vi "Main.vi"() -> ()   [LabVIEW 2020, in "ChromTech Next Gen Compensator Pump.lvlib"]
uses:
  ChromTech Next Gen Compensator Pump.lvlib
  process loops/Instrument Manager/Instrument State.ctl
  process loops/UI Manager/Data Display Loop Data.ctl
  process loops/Logging/Logging Configuration.ctl
  process loops/UI Manager/UI Data.ctl
  process loops/UI Manager/UI Display State.ctl
  Typedefs/System Control Data.ctl
  <vilib>/Utility/error.llb/Error Cluster From Error Code.vi
  <vilib>/ErrorRing/Error Ring.xnode
  support/Message Queue/Message Queue.lvlib
  support/User Event - Stop/User Event - Stop.lvlib
  process loops/Instrument Manager/Instrument Manager.lvlib
  process loops/Acquisition/Acquisition.lvlib
  process loops/Remote Connection Manager/Remote Connection Manager.lvlib
  process loops/Logging/Logging.lvlib
panel:
  in  "This Flow Rate (mL/min)":dbl format="%.3f"
  in  "Total Flow (mL/min)":dbl=0.1 format="%.3f"
  in  "Time Interval (sec)":i32=1200
  out "Data Graph":cluster{timestamp[], dbl[]}[](graph)
  in  "Config Log Btn":bool
  in  "Sampling rate\n(sec/sample)":dbl=5.0 min=0.1 step=0.1
  in  "Log Data":bool
  in  "Stop Btn":bool=TRUE
  in  "Run Btn":bool
  out "Data Ind":dbl format="%d psi"
  in  "Other Flow Rate (mL/min)":dbl format="%.3f"
  out "VISA resource":refnum<visa-resource-name>
  # "Pump Control Panel"
  # "Config"
  # "Pump Control"
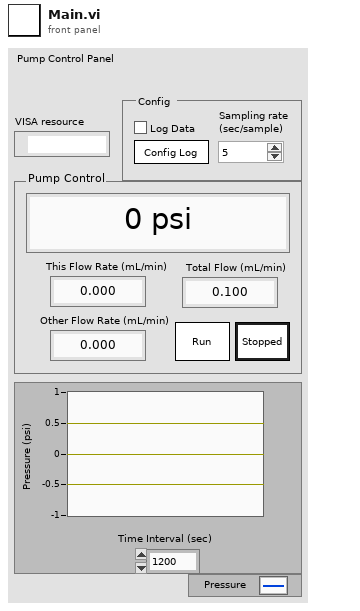
[diagram p1: front panel]
types:
  T1 = typedef "ChromTech Next Gen Compensator Pump.lvlib/Data Display Loop Data.ctl" = cluster{"Data Timestamps":timestamp[], "Data Values":dbl[], "Previous Run State":bool}
  T2 = typedef "ChromTech Next Gen Compensator Pump.lvlib/Instrument Manager.lvlib/Instrument State.ctl" = cluster{"VISA Resource":refnum<visa-resource-name>, "Flow Rate":dbl, "Running":bool, "Running Since":timestamp, "Pressure Data Point":cluster{"Time Stamp":timestamp, "Value":dbl}, "Upper Pressure Fault":bool, "Lower Pressure Fault":bool, "Motor Stall Fault":bool, "Sampling Rate (sec/sample)":dbl, "Retry Attempts":i32, "Fast Comms":bool, "Total Flow Rate":dbl, "Other Flow Rate":dbl}
  T3 = typedef "ChromTech Next Gen Compensator Pump.lvlib/Message Queue.lvlib/All Message Queues.ctl" = cluster{"System Control":refnum<queue>, "Instrument":refnum<queue>, "Remote":refnum<queue>, "UI":refnum<queue>, "Acquisition":refnum<queue>, "Logging":refnum<queue>}
  T4 = typedef "ChromTech Next Gen Compensator Pump.lvlib/UI Display State.ctl" = enum16{"Shown", "Hidden"}
  T5 = enum8{"Enabled", "Disabled", "Disabled and Grayed Out"}
  T6 = typedef "ChromTech Next Gen Compensator Pump.lvlib/UI Data.ctl" = cluster{"VISA Resource Ind":refnum<vi>, "Setpoint Ctl":refnum<vi>, "Run Btn":refnum<vi>, "Stop Btn":refnum<vi>, "Data Ind":refnum<vi>, "Log Data":refnum<vi>, "Config Log Btn":refnum<vi>, "Sampling rate\n(sec/sample)":refnum<vi>, "Data Graph":refnum<vi>, "This Flow Rate (mL/min)":refnum<vi>, "Other Flow Rate (mL/min)":refnum<vi>, "Total Flow (mL/min)":refnum<vi>}
  T7 = typedef "ChromTech Next Gen Compensator Pump.lvlib/Logging.lvlib/Logging Configuration.ctl" = cluster{"Log Directory Path":path, "Log File Path":path, "Log File Prefix":string, "Log File Extension":string, "File Delimiter":string, "Header Info":string[][], "Channels":string[], "Log Instrument Runs":bool}
  T8 = typedef "ChromTech Next Gen Compensator Pump.lvlib/System Control Data.ctl" = cluster{"Example Value <Replace Me>":dbl, "Log Runs":bool, "Clone":bool}
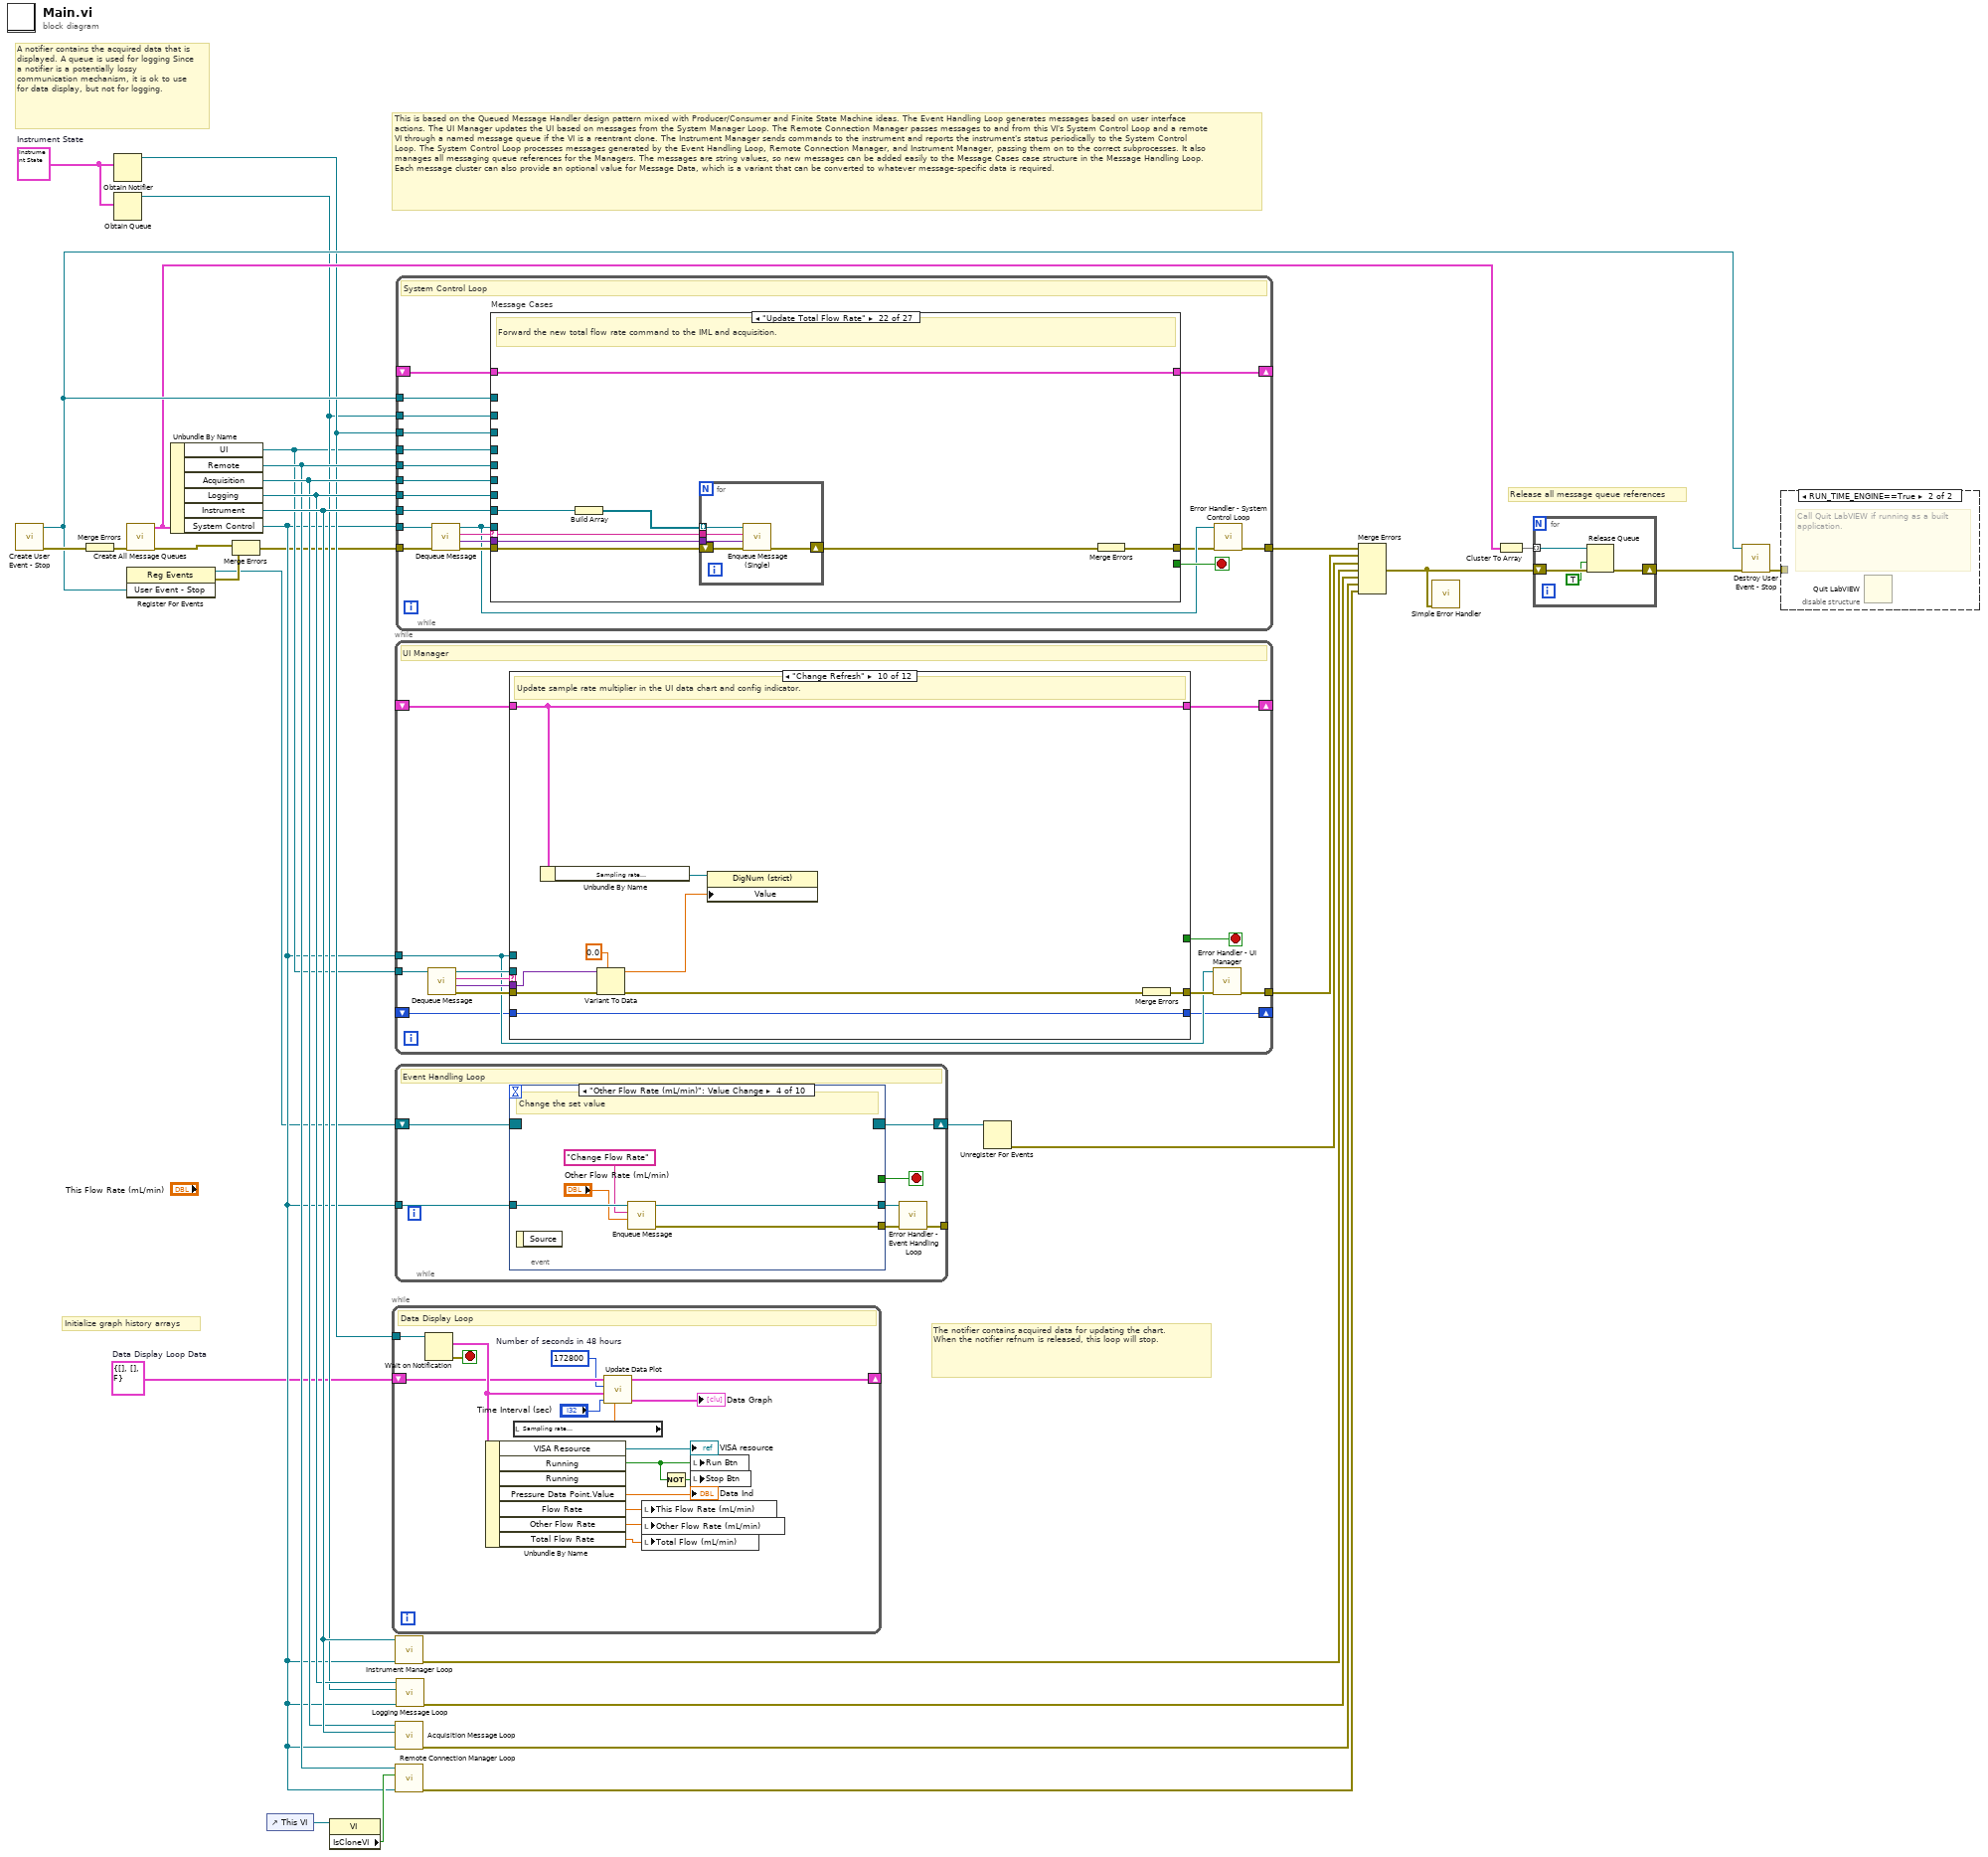
[diagram p0: block diagram]
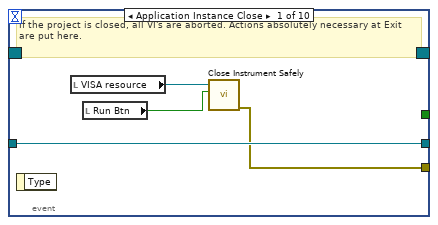
[diagram p2: hidden frame]
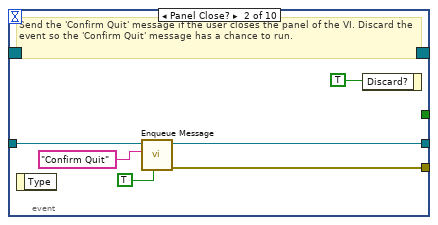
[diagram p3: hidden frame]
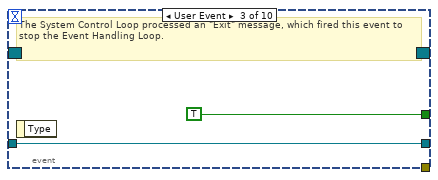
[diagram p4: hidden frame]
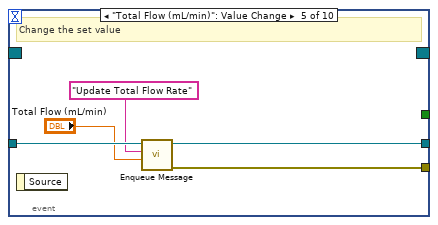
[diagram p5: hidden frame]
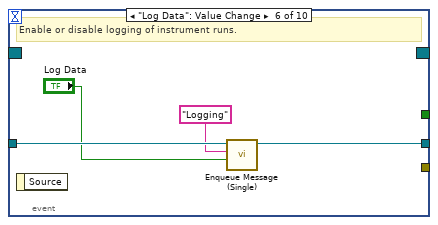
[diagram p6: hidden frame]
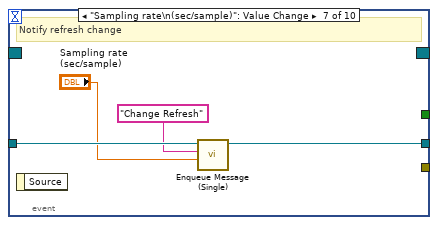
[diagram p7: hidden frame]
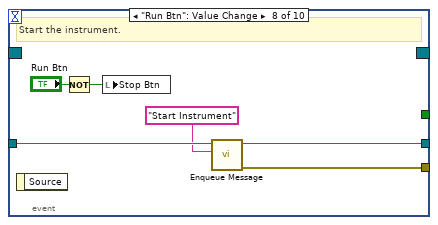
[diagram p8: hidden frame]
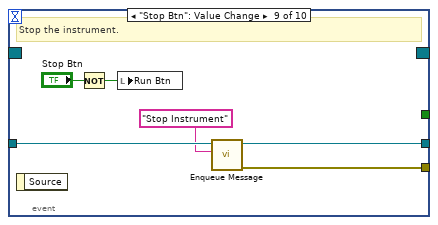
[diagram p9: hidden frame]
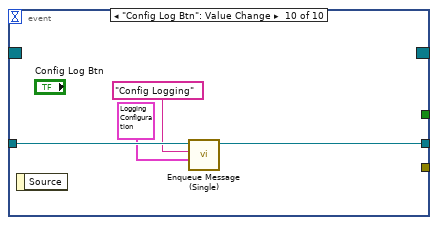
[diagram p10: hidden frame]
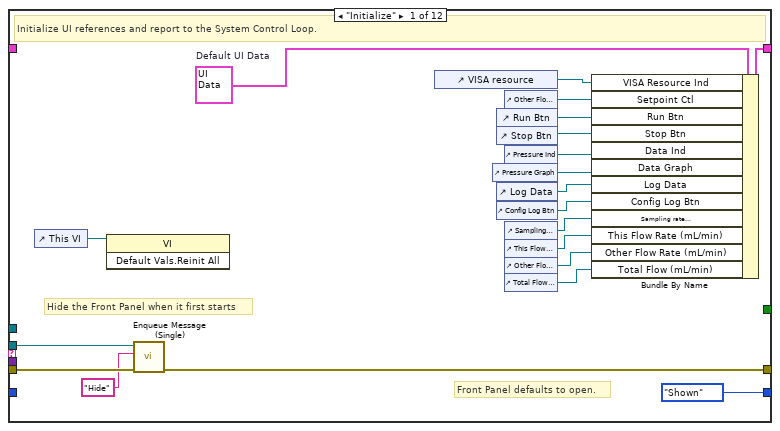
[diagram p11: hidden frame]
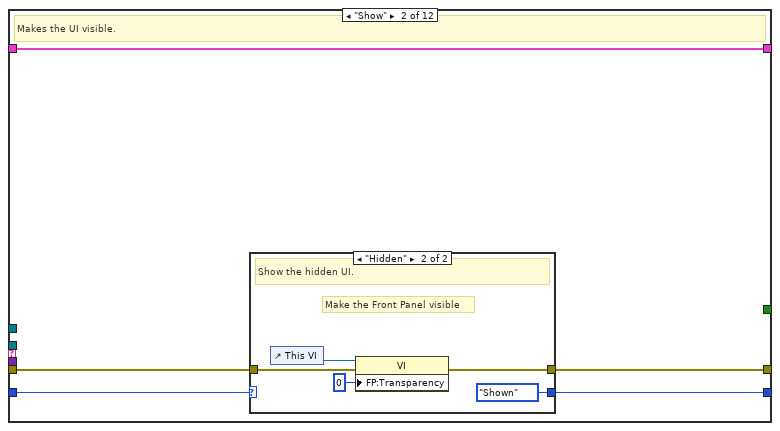
[diagram p12: hidden frame]
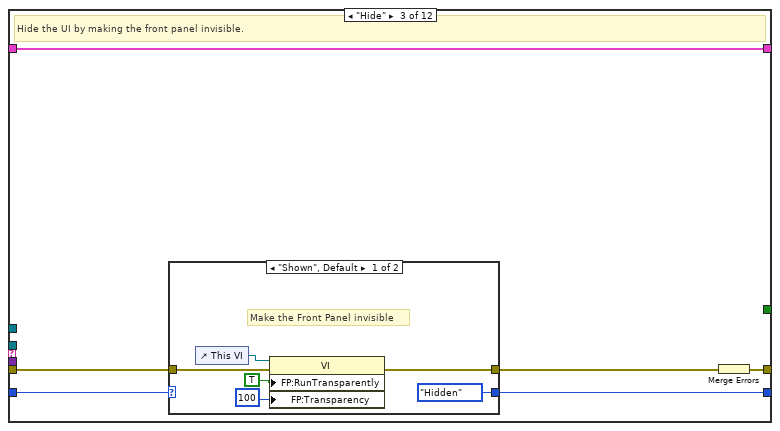
[diagram p14: hidden frame]
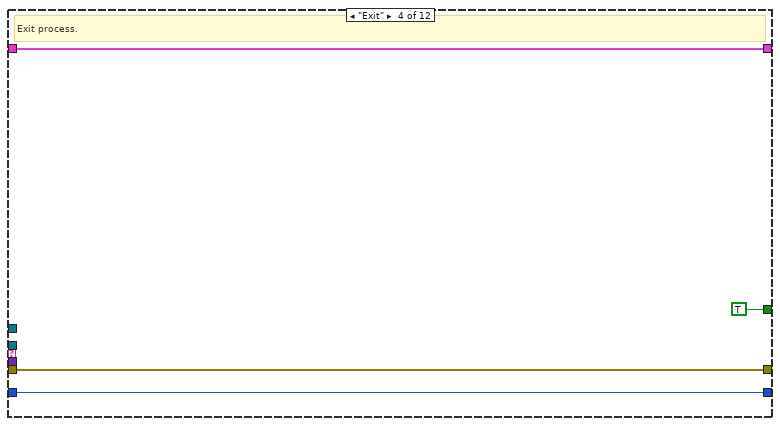
[diagram p16: hidden frame]
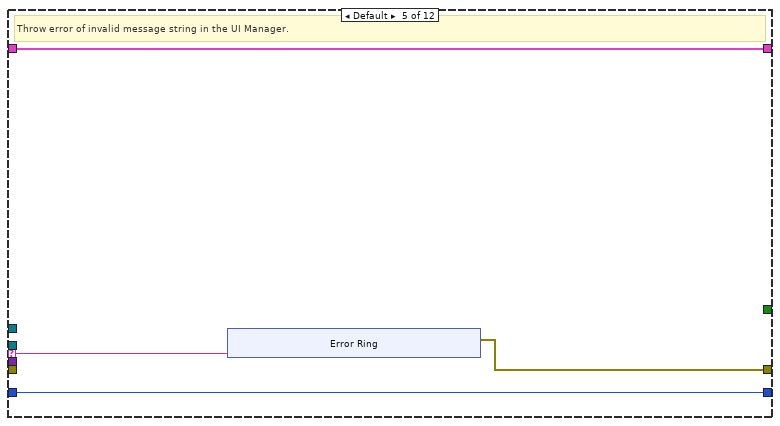
[diagram p17: hidden frame]
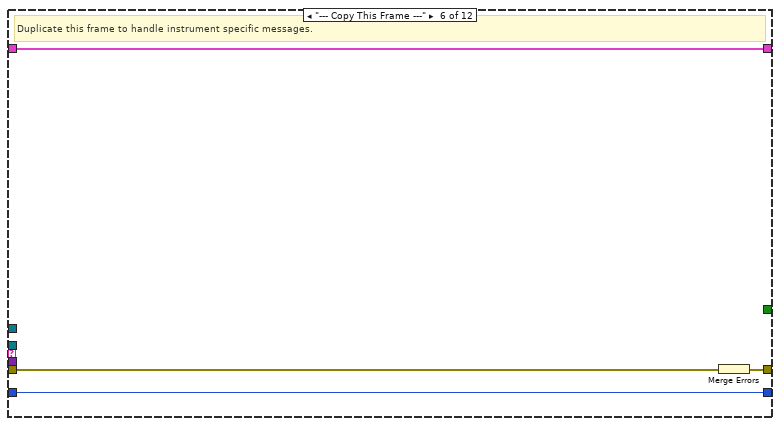
[diagram p18: hidden frame]
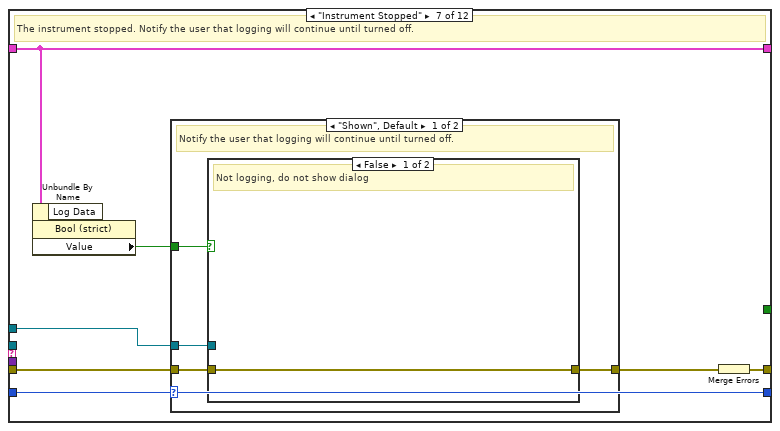
[diagram p19: hidden frame]
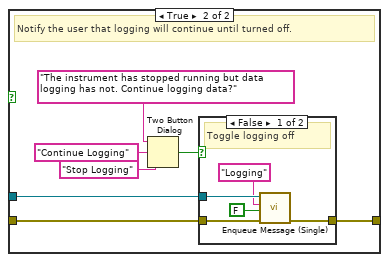
[diagram p20: hidden frame]
diagram:
  w1 = T1 {"Data Timestamps"=[], "Data Values"=[], "Previous Run State"=FALSE}  # Data Display Loop Data
  w7 = T2 {"VISA Resource"="", "Flow Rate"=0.0, "Running"=FALSE, "Running Since"=timestamp(0 s since 1904-01-01), "Pressure Data Point"={"Time Stamp"=timestamp(0 s since 1904-01-01), "Value"=0.0}, "Upper Pressure Fault"=FALSE, "Lower Pressure Fault"=FALSE, "Motor Stall Fault"=FALSE, "Sampling Rate (sec/sample)"=0.0, "Retry Attempts"=0, "Fast Comms"=FALSE, "Total Flow Rate"=0.0, "Other Flow Rate"=0.0}  # Instrument State
  # "Initialize graph history arrays"
  # "A notifier contains the acquired data that is displayed. A queue is used for logging Since a notifier is a potentially lossy communication mechanism, it is ok to use for data display, but not for logging."
  # "The notifier contains acquired data for updating the chart. When the notifier refnum is released, this loop will stop."
  # "Release all message queue references"
  # "This is based on the Queued Message Handler design pattern mixed with Producer/Consumer and Finite State Machine ideas. The Event Handling Loop generates messages based on user interface actions. The UI Manager updates the UI based on messages from the System Manager Loop. The Remote Connection Manager passes messages to and from this VI's System Control Loop and a remote VI through a named message queue if the VI is a reentrant clone. The Instrument Manager sends commands to the instrument and reports the instrument's status periodically to the System Control Loop. The System Control Loop processes messages generated by the Event Handling Loop, Remote Connection Manager, and Instrument Manager, passing them on to the correct subprocesses. It also manages all messaging queue references for the Managers. The messages are string values, so new messages can be added easily to the Message Cases case structure in the Message Handling Loop.  Each message cluster can also provide an optional value for Message Data, which is a variant that can be converted to whatever message-specific data is required."
  n1 = call "Create User Event - Stop.vi"() -> ("error out"=w26:errorcluster, "User Event - Stop"=w22:refnum<user-event>)  [unwired: 10 in]
  n2 = Merge Errors(w26) -> (w25:errorcluster)
  n3 = Obtain Notifier(notification data type=w7) -> (notifier out=w8:refnum<notifier>)  [unwired: 3 in, 2 out]
  n4 = Obtain Queue(element data type=w7) -> (queue out=w6:refnum<queue>)  [unwired: 4 in, 2 out]
  n5 = call "Create All Message Queues.vi"("error in (no error)"=w25) -> ("error out"=w28:errorcluster, "Message Queues out"=w11:T3)  [unwired: 9 in]
  n6 = register-events(w22) -> (reference out=w2:refnum<event-registration>, error out=w13:errorcluster)  [unwired: 2 in]
  n7 = Unbundle By Name(w11) -> ("UI"=w5:refnum<queue>, "Remote"=w29:refnum<queue>, "Acquisition"=w30:refnum<queue>, "Logging"=w31:refnum<queue>, "Instrument"=w32:refnum<queue>, "System Control"=w4:refnum<queue>)
  n8 = Merge Errors(w28, w13) -> (w3:errorcluster)
  n9 = control-ref of="This VI"() -> (w21:refnum<vi>)
  n10 = property class="VI"(reference=w21) -> ("IsCloneVI"=w20:bool)  [unwired: 1 in, 2 out]
  n11 = while "Data Display Loop" {
    tunnel: w8 -> [w48]
    shift-right: [w39] -> _
    shift-left: w1 -> [w40]
    stop <- w47 stop-if-true
    w36 = 172800  # Number of seconds in 48 hours
    # "Data Display Loop"
    n12 = Wait on Notification(notifier=w48) -> (notification=w41:T2, error out=w47:errorcluster)  [unwired: 3 in, 2 out]
    n13 = Unbundle By Name(w41) -> ("VISA Resource"=→"VISA resource":refnum<visa-resource-name>, "Running"=w45:bool, "Pressure Data Point.Value"=→"Data Ind":dbl, "Flow Rate"=w35:dbl, "Other Flow Rate"=w34:dbl, "Total Flow Rate"=w33:dbl)  [unwired: 1 out]
    n14 = local read "Sampling rate\n(sec/sample)"() -> (w37:dbl)
    n15 = call "Update Data Plot.vi"("Sample Rate (sec/sample)"=w37, "Time interval (s)"="Time Interval (sec)", "Instrument State"=w41, "History length (-1; unlimited)"=w36, "Graph History Arrays in"=w40) -> ("Updated Plot History"=→"Data Graph":cluster{timestamp[], dbl[]}[], "Graph History Arrays out"=w39:T1)  [unwired: 5 in]
    n16 = local write "This Flow Rate (mL/min)"(w35) -> ()
    n17 = local write "Other Flow Rate (mL/min)"(w34) -> ()
    n18 = local write "Total Flow (mL/min)"(w33) -> ()
    n19 = Not(x=w45) -> (.not. x?=w44:bool)
    n20 = local write "Run Btn"(w45) -> ()
    n21 = local write "Stop Btn"(w44) -> ()
  }
  n22 = while {
    tunnel: w5 -> [w61]
    tunnel: w4 -> [w52]
    tunnel: [w53] -> w19
    shift-right: [w56] -> _
    shift-left: _ -> [w55]
    shift-right: [w50] -> _
    shift-left: _ -> [w49]
    stop <- w51 stop-if-true
    # "UI Manager"
    n23 = call "Dequeue Message.vi"("Message Queue"=w61) -> ("error out"=w59:errorcluster, "Message Data"=w57:variant, "Message"=w58:string, "dup Message Queue"=w60:refnum<queue>)  [unwired: 7 in]
    n24 = case shown="\"Change Refresh\"" w58 {
      selector: w58 -> [_ _ _ _ w115 _ _ _ _ _ _ _]
      tunnel: w60 -> [w72 _ _ _ _ _ _ _ _ _ _ _]
      tunnel: w59 -> [w78 w85 w97 w111 _ w124 w132 w160 w168 w171 w192 w203]
      tunnel: w57 -> [_ _ _ _ _ _ _ _ _ w177 w190 w202]
      tunnel: w52 -> [_ _ _ _ _ _ w130 _ _ _ _ _]
      tunnel: [w73 w84 w98 w111 w114 w125 w134 w161 w169 w178 w193 w204] -> w54
      tunnel: [w80 w86 w99 w110 w113 w126 w129 w156 w162 w173 w185 w198] -> w56
      tunnel: w55 -> [_ w86 w99 w110 w113 w126 w129 w156 w162 w173 w185 w198]
      tunnel: [_ _ _ TRUE _ _ _ _ _ _ _ _] -> w51
      tunnel: w49 -> [_ w83 w95 w108 w112 w123 w133 w159 w167 w175 w186 w199]
      tunnel: [UI_Display_State."Shown" ("UI Display State") w82 w94 w108 w112 w123 w133 w159 w167 w175 w186 w199] -> w50
      frame "Initialize" {
        w81 = T6 {"VISA Resource Ind"=refnum, "Setpoint Ctl"=refnum, "Run Btn"=refnum, "Stop Btn"=refnum, "Data Ind"=refnum, "Log Data"=refnum, "Config Log Btn"=refnum, "Sampling rate\n(sec/sample)"=refnum, "Data Graph"=refnum, "This Flow Rate (mL/min)"=refnum, "Other Flow Rate (mL/min)"=refnum, "Total Flow (mL/min)"=refnum}  # Default UI Data
        # "Front Panel defaults to open."
        # "Hide the Front Panel when it first starts"
        # "Initialize UI references and report to the System Control Loop."
        n25 = control-ref of="This VI"() -> (w65:refnum<vi>)
        n26 = invoke class="VI" method="Default Vals.Reinit All"(reference=w65) -> ()  [unwired: 2 in, 3 out]
        n27 = call "Enqueue Message (Single).vi"("error in (no error)"=w78, "Message"="Hide", "Message Queue"=w72) -> ("error out"=w73:errorcluster)  [unwired: 7 in, 1 out]
        n28 = control-ref of="VISA resource"() -> (w77:refnum<vi>)
        n29 = control-ref of="Pressure Graph"() -> (w69:refnum<vi>)
        n30 = control-ref of="Run Btn"() -> (w75:refnum<vi>)
        n31 = control-ref of="Stop Btn"() -> (w76:refnum<vi>)
        n32 = control-ref of="Log Data"() -> (w68:refnum<vi>)
        n33 = control-ref of="Config Log Btn"() -> (w67:refnum<vi>)
        n34 = control-ref of="Other Flow Rate (mL/min)"() -> (w79:refnum<vi>)
        n35 = control-ref of="Pressure Ind"() -> (w74:refnum<vi>)
        n36 = control-ref of="Sampling rate (sec/sample)"() -> (w66:refnum<vi>)
        n37 = control-ref of="This Flow Rate (mL/min)"() -> (w64:refnum<vi>)
        n38 = control-ref of="Other Flow Rate (mL/min)"() -> (w62:refnum<vi>)
        n39 = control-ref of="Total Flow (mL/min)"() -> (w63:refnum<vi>)
        n40 = Bundle By Name(cluster=w81, "VISA Resource Ind"=w77, "Setpoint Ctl"=w79, "Run Btn"=w75, "Stop Btn"=w76, "Data Ind"=w74, "Data Graph"=w69, "Log Data"=w68, "Config Log Btn"=w67, "Sampling rate\n(sec/sample)"=w66, "This Flow Rate (mL/min)"=w64, "Other Flow Rate (mL/min)"=w62, "Total Flow (mL/min)"=w63) -> (w80:T6)
      }
      frame "Show" {
        # "Makes the UI visible."
        n41 = case shown="\"Hidden\"" w83 {
          selector: w83 -> [w88 _]
          tunnel: w85 -> [w87 w93]
          tunnel: [w87 w91] -> w84
          tunnel: [w88 UI_Display_State."Shown" ("UI Display State")] -> w82
          frame "Shown", Default {
            # "Do nothing if UI is already shown."
          }
          frame "Hidden" {
            # "Make the Front Panel visible"
            # "Show the hidden UI."
            n42 = control-ref of="This VI"() -> (w92:refnum<vi>)
            n43 = property class="VI"(reference=w92, error in=w93, "FP:Transparency"=u8 0 ("Front Panel Window:Transparency")) -> (error out=w91:errorcluster)  [unwired: 1 out]
          }
        }
      }
      frame "Hide" {
        # "Hide the UI by making the front panel invisible."
        n44 = case shown="\"Shown\", Default" w95 {
          selector: w95 -> [_ w107]
          tunnel: w97 -> [w102 w106]
          tunnel: [w101 w106] -> w96
          tunnel: [UI_Display_State."Hidden" ("UI Display State") w107] -> w94
          frame "Shown", Default {
            # "Make the Front Panel invisible"
            n45 = control-ref of="This VI"() -> (w105:refnum<vi>)
            n46 = property class="VI"(reference=w105, error in=w102, "FP:RunTransparently"=TRUE ("Front Panel Window:Run VI Transparently"), "FP:Transparency"=u8 100 ("Front Panel Window:Transparency")) -> (error out=w101:errorcluster)  [unwired: 1 out]
          }
          frame "Hidden" {
          }
        }
        n47 = Merge Errors(w96) -> (w98:errorcluster)
      }
      frame "Exit" {
        # "Exit process."
      }
      frame Default {
        # "Throw error of invalid message string in the UI Manager."
        n48 = xnode "Error Ring"("parameter 0"=w115) -> ("error out"=w114:errorcluster)
      }
      frame "--- Copy This Frame ---" {
        # "Duplicate this frame to handle instrument specific messages."
        n49 = Merge Errors(w124) -> (w125:errorcluster)
      }
      frame "Instrument Stopped" {
        # "The instrument stopped. Notify the user that logging will continue until turned off."
        n50 = Unbundle By Name(w129) -> ("Log Data"=w128:refnum<vi>)
        n51 = property class="Bool (strict)"(reference=w128) -> ("Value"=w127:bool)  [unwired: 1 in, 2 out]
        n52 = case shown="\"Shown\", Default" w133 {
          tunnel: w132 -> [w138 w153]
          tunnel: [w137 w153] -> w131
          tunnel: w130 -> [w136 _]
          tunnel: w127 -> [w135 _]
          frame "Shown", Default {
            # "Notify the user that logging will continue until turned off."
            n53 = case shown="False" w135 {
              tunnel: w138 -> [w139 w142]
              tunnel: [w139 w141] -> w137
              tunnel: w136 -> [_ w140]
              frame False {
                # "Not logging, do not show dialog"
              }
              frame True {
                # "Notify the user that logging will continue until turned off."
                n54 = Two Button Dialog(message="The instrument has stopped running but data logging has not. Continue logging data?", 1:"Stop Logging" ("F button name (\"Cancel\")"), 2:"Continue Logging" ("T button name (\"OK\")")) -> (T button?=w143:bool)
                n55 = case shown="False" w143 {
                  tunnel: w142 -> [w151 w152]
                  tunnel: [w150 w152] -> w141
                  tunnel: w140 -> [w149 _]
                  frame False {
                    # "Toggle logging off"
                    n56 = call "Enqueue Message (Single).vi"("error in (no error)"=w151, "Message Data"=FALSE, "Message"="Logging", "Message Queue"=w149) -> ("error out"=w150:errorcluster)  [unwired: 6 in, 1 out]
                  }
                  frame True {
                    # "Continues logging. Do nothing more"
                  }
                }
              }
            }
          }
          frame "Hidden" {
            # "Hidden, do not show dialog"
          }
        }
        n57 = Merge Errors(w131) -> (w134:errorcluster)
      }
      frame "Logging Started" {
        # "Indicate that logging started."
        n58 = Unbundle By Name(w156) -> ("Log Data"=w158:refnum<vi>)
        n59 = property class="Bool (strict)"(reference=w158, "Value"=TRUE ("Log Data")) -> ()  [unwired: 1 in, 2 out]
        n60 = Unbundle By Name(w156) -> ("Config Log Btn"=w155:refnum<vi>)
        n61 = property class="Bool"(reference=w155, "DisabledEnum"=T5."Disabled and Grayed Out" ("Disabled")) -> ()  [unwired: 1 in, 2 out]
        n62 = Merge Errors(w160) -> (w161:errorcluster)
      }
      frame "Logging Stopped" {
        # "Indicate that logging stopped."
        n63 = Unbundle By Name(w162) -> ("Log Data"=w166:refnum<vi>)
        n64 = property class="Bool (strict)"(reference=w166, "Value"=FALSE ("Log Data")) -> ()  [unwired: 1 in, 2 out]
        n65 = Unbundle By Name(w162) -> ("Config Log Btn"=w164:refnum<vi>)
        n66 = property class="Bool"(reference=w164, "DisabledEnum"=T5."Enabled" ("Disabled")) -> ()  [unwired: 1 in, 2 out]
        n67 = Merge Errors(w168) -> (w169:errorcluster)
      }
      frame "Change Refresh" {
        # "Update sample rate multiplier in the UI data chart and config indicator."
        n68 = Unbundle By Name(w173) -> ("Sampling rate\n(sec/sample)"=w174:refnum<vi>)
        n69 = Variant To Data(error in=w171, type=0.0, Variant=w177) -> (data=w172:dbl, error out=w170:errorcluster)
        n70 = property class="DigNum (strict)"(reference=w174, "Value"=w172) -> ()  [unwired: 1 in, 2 out]
        n71 = Merge Errors(w170) -> (w178:errorcluster)
      }
      frame "Update Pressure Units" {
        # "Change the units of the display."
        n72 = Variant To Data(type="", Variant=w190) -> (data=w180:string)  [unwired: 1 in, 1 out]
        n73 = call <vilib>:"Space Constant.vi"() -> ("String"=w189:string)
        n74 = Concatenate Strings("%d" ("string"), w189, w180) -> (w187:string)
        n75 = Unbundle By Name(w185) -> ("Data Ind"=w184:refnum<vi>, "Data Graph"=w179:refnum<vi>)
        n76 = Concatenate Strings("Pressure (" ("concatenated string"), w180, ")" ("string")) -> (w183:string)
        n77 = property on="Property Node" class="DigNum (strict)"(reference=w184, "FormatString"=w187) -> ()  [unwired: 1 in, 2 out]
        n78 = property class="XYGraph (strict)"(reference=w179, "YScale.NameLbl.Text"=w183) -> ()  [unwired: 1 in, 2 out]
        n79 = Merge Errors(w192) -> (w193:errorcluster)
      }
      frame "Update Flow Rate Units" {
        # "Change the units of the setpoint display."
        n80 = Variant To Data(type="", Variant=w202) -> (data=w196:string)  [unwired: 1 in, 1 out]
        n81 = Concatenate Strings("Flow Rate (" ("string"), w196, ")" ("string")) -> (w200:string)
        n82 = Unbundle By Name(w198) -> ("Setpoint Ctl"=w197:refnum<vi>)
        n83 = property on="Property Node" class="DigNum (strict)"(reference=w197, "FormatString"=w200) -> ()  [unwired: 1 in, 2 out]
        n84 = Merge Errors(w203) -> (w204:errorcluster)
      }
    }
    n85 = call "Error Handler - UI Manager.vi"("error in (no error)"=w54, "Message Queue"=w52) -> ("dup error in"=w53:errorcluster)  [unwired: 8 in, 1 out]
  }
  n86 = while {
    tunnel: w4 -> [w211]
    shift-right: [w209] -> w23
    shift-left: w2 -> [w210]
    tunnel: [w205] -> _
    stop <- w207 stop-if-true
    # "Event Handling Loop"
    n87 = event shown="[3] \"Other Flow Rate (mL/min)\": Value Change" {
      selector: w210 -> [_ _ _ _ _ _ _ _ _ _]
      dyn-events: [_ _ _ _ _ _ _ _ _ _] -> w209
      timeout: _ -> [_ _ _ _ _ _ _ _ _ _]
      tunnel: [_ _ TRUE ("Discard?") _ _ _ _ _ _ _] -> w207
      tunnel: w211 -> [w215 w220 w223 w228 w233 w237 w241 w247 w253 w257]
      tunnel: [w214 w219 _ w225 w230 _ _ w245 w251 _] -> w208
      tunnel: [w215 w218 w223 w227 w232 w236 w240 w246 w252 w256] -> w206
      event Application Instance Close {
        # "If the project is closed, all VI's are aborted. Actions absolutely necessary at Exit are put here."
        n88 = event-data() -> ()  [unwired: 1 in, 1 out]
        n89 = local read "VISA resource"() -> (w213:refnum<visa-resource-name>)
        n90 = local read "Run Btn"() -> (w212:bool)
        n91 = call "Close Instrument Safely.vi"("Running (F)"=w212, "VISA Refnum in"=w213) -> ("error out"=w214:errorcluster)  [unwired: 9 in]
      }
      event Panel Close? {
        # "Send the 'Confirm Quit' message if the user closes the panel of the VI. Discard the event so the 'Confirm Quit' message has a chance to run."
        n92 = event-data() -> ()  [unwired: 1 in, 1 out]
        n93 = call-poly "Enqueue Message.vi"("Priority Message? (F)"=TRUE, "Message"="Confirm Quit", "Message Queue"=w220) -> ("error out"=w219:errorcluster, "dup Message Queue"=w218:refnum<queue>)  [unwired: 7 in]
        n94 = event-data("Discard?"=TRUE) -> ()  [unwired: 1 in, 1 out]
      }
      event User Event {
        # "The System Control Loop processed an \"Exit\" message, which fired this event to stop the Event Handling Loop."
        n95 = event-data() -> ()  [unwired: 1 in, 1 out]
      }
      event "Other Flow Rate (mL/min)": Value Change {
        # "Change the set value"
        n96 = event-data() -> ()  [unwired: 1 in, 1 out]
        n97 = call-poly "Enqueue Message.vi"("Message Data"="Other Flow Rate (mL/min)", "Message"="Change Flow Rate", "Message Queue"=w228) -> ("error out"=w225:errorcluster, "dup Message Queue"=w227:refnum<queue>)  [unwired: 7 in]
      }
      event "Total Flow (mL/min)": Value Change {
        # "Change the set value"
        n98 = event-data() -> ()  [unwired: 1 in, 1 out]
        n99 = call-poly "Enqueue Message.vi"("Message Data"="Total Flow (mL/min)", "Message"="Update Total Flow Rate", "Message Queue"=w233) -> ("error out"=w230:errorcluster, "dup Message Queue"=w232:refnum<queue>)  [unwired: 7 in]
      }
      event "Log Data": Value Change {
        # "Enable or disable logging of instrument runs."
        n100 = event-data() -> ()  [unwired: 1 in, 1 out]
        n101 = call "Enqueue Message (Single).vi"("Message Data"="Log Data", "Message"="Logging", "Message Queue"=w237) -> ("dup Message Queue"=w236:refnum<queue>)  [unwired: 7 in, 1 out]
      }
      event "Sampling rate\n(sec/sample)": Value Change {
        # "Notify refresh change"
        n102 = event-data() -> ()  [unwired: 1 in, 1 out]
        n103 = call "Enqueue Message (Single).vi"("Message Data"="Sampling rate\n(sec/sample)", "Message"="Change Refresh", "Message Queue"=w241) -> ("dup Message Queue"=w240:refnum<queue>)  [unwired: 7 in, 1 out]
      }
      event "Run Btn": Value Change {
        # "Start the instrument."
        n104 = event-data() -> ()  [unwired: 1 in, 1 out]
        n105 = Not(x="Run Btn") -> (.not. x?=w242:bool)
        n106 = local write "Stop Btn"(w242) -> ()
        n107 = call-poly "Enqueue Message.vi"("Message"="Start Instrument", "Message Queue"=w247) -> ("error out"=w245:errorcluster, "dup Message Queue"=w246:refnum<queue>)  [unwired: 8 in]
      }
      event "Stop Btn": Value Change {
        # "Stop the instrument."
        n108 = event-data() -> ()  [unwired: 1 in, 1 out]
        n109 = Not(x="Stop Btn") -> (.not. x?=w248:bool)
        n110 = local write "Run Btn"(w248) -> ()
        n111 = call-poly "Enqueue Message.vi"("Message"="Stop Instrument", "Message Queue"=w253) -> ("error out"=w251:errorcluster, "dup Message Queue"=w252:refnum<queue>)  [unwired: 8 in]
      }
      event "Config Log Btn": Value Change {
        n112 = event-data() -> ()  [unwired: 1 in, 1 out]
        n113 = call "Enqueue Message (Single).vi"("Message Data"=T7 {"Log Directory Path"=path "", "Log File Path"=path "", "Log File Prefix"="Experiment", "Log File Extension"="csv", "File Delimiter"=",", "Header Info"=[], "Channels"=[], "Log Instrument Runs"=FALSE} ("Logging Configuration"), "Message"="Config Logging", "Message Queue"=w257) -> ("dup Message Queue"=w256:refnum<queue>)  [unwired: 7 in, 1 out]
      }
    }
    n114 = call "Error Handler - Event Handling Loop.vi"("error in (no error)"=w208, "Message Queue"=w206) -> ("dup error in"=w205:errorcluster)  [unwired: 8 in, 1 out]
  }
  n115 = call "Instrument Manager Loop.vi"("System Control"=w4, "Instrument Manager"=w32) -> ("error out"=w17:errorcluster)  [unwired: 9 in]
  n116 = call "Acquisition Message Loop.vi"("System Control"=w4, "Instrument Manager"=w32, "Acquisition"=w30) -> ("error out"=w15:errorcluster)  [unwired: 8 in]
  n117 = call "Remote Connection Manager Loop.vi"("System Control"=w4, "IsCloneVI (false)"=w20, "Remote"=w29) -> ("error out"=w14:errorcluster)  [unwired: 8 in]
  n118 = while {
    tunnel: w4 -> [w268]
    shift-right: [w275] -> _
    shift-left: _ -> [w276]
    tunnel: w22 -> [w273]
    tunnel: w3 -> [w272]
    tunnel: [w266] -> w27
    tunnel: w32 -> [w264]
    tunnel: w29 -> [w263]
    tunnel: w5 -> [w262]
    tunnel: w30 -> [w261]
    tunnel: w31 -> [w260]
    tunnel: w8 -> [w259]
    tunnel: w6 -> [w258]
    stop <- w274 stop-if-true
    # "System Control Loop"
    n119 = call "Dequeue Message.vi"("error in (no error)"=w272, "Message Queue"=w268) -> ("error out"=w271:errorcluster, "Message Data"=w269:variant, "Message"=w270:string, "dup Message Queue"=w267:refnum<queue>)  [unwired: 6 in]
    n120 = case "Message Cases" shown="\"Update Total Flow Rate\"" w270 {
      selector: w270 -> [_ _ _ w318 w331 w342 w362 w377 w390 w404 w410 _ w456 w463 w470 w477 w484 w494 w508 w523 w537 w550 w561 w568 w578 w593 w615]
      tunnel: w267 -> [_ _ w298 _ _ _ _ _ _ _ _ _ _ _ _ _ _ _ _ _ _ _ _ _ _ _ _]
      tunnel: w271 -> [w280 w295 w302 _ _ w345 w365 w380 w393 w408 w426 w439 w460 w467 w474 w481 w488 w497 w511 w527 w541 w554 w564 w571 _ _ _]
      tunnel: [w279 w289 w300 w321 w332 w351 w366 w381 w395 w409 w417 w444 w461 w468 w475 w482 w489 w498 w512 w525 w539 w552 w565 w572 w577 w592 w614] -> w265
      tunnel: w276 -> [_ w294 w301 w317 w333 w352 w367 w382 w396 w407 w416 w445 w462 w469 w476 w483 w490 w499 w513 w526 w540 w553 w566 w573 w576 w589 w612]
      tunnel: [w281 w294 w301 w317 w333 w352 w367 w382 w396 w407 w416 w443 w462 w469 w476 w483 w490 w499 w513 w526 w540 w553 w566 w573 w576 w589 w612] -> w275
      tunnel: [_ _ _ TRUE _ _ _ _ _ _ _ _ _ _ _ _ _ _ _ _ _ _ _ _ _ _ _] -> w274
      tunnel: w269 -> [_ w293 _ w322 _ w341 w361 w376 w389 w403 w411 w441 w457 w464 w471 w478 w485 w495 w509 w522 w536 w549 w562 w569 w579 w594 w610]
      tunnel: w273 -> [_ _ _ w319 _ _ _ _ _ _ _ _ _ _ _ _ _ _ _ _ _ _ _ _ _ _ _]
      tunnel: w264 -> [w278 _ _ w314 _ w346 _ _ _ w405 _ _ _ _ _ _ _ _ _ _ w535 w548 w560 w567 _ _ _]
      tunnel: w263 -> [_ _ _ w313 _ w349 _ _ w394 _ w421 _ _ _ _ _ _ w493 w507 _ _ _ _ _ w580 w590 w613]
      tunnel: w262 -> [_ _ _ w312 _ w348 w359 w374 _ _ w420 _ _ _ _ _ _ w492 w506 w520 _ _ _ _ _ w588 _]
      tunnel: w261 -> [_ _ _ w316 _ w350 _ _ _ _ w423 _ _ _ _ _ _ _ _ w521 w534 _ _ _ w575 _ _]
      tunnel: w260 -> [_ _ _ w315 _ w347 w360 w375 _ _ w413 w437 w458 w465 w472 w479 w486 _ _ _ _ _ _ _ w574 _ _]
      tunnel: w259 -> [_ _ _ w309 _ _ _ _ _ _ _ _ _ _ _ _ _ _ _ _ _ _ _ _ _ _ w611]
      tunnel: w258 -> [_ _ _ w307 _ _ _ _ _ _ _ _ _ _ _ _ _ _ _ _ _ _ _ _ _ _ w607]
      frame "Initialize" {
        w282 = T8 {"Example Value <Replace Me>"=0.0, "Log Runs"=FALSE, "Clone"=FALSE}  # Default Data
        # "Initialize the system control loop and system."
        n121 = control-ref of="This VI"() -> ()  [unwired: 1 out]
        n122 = property on="Property Node" class="VI"() -> ("IsCloneVI"=w277:bool)  [unwired: 2 in, 2 out]
        n123 = Bundle By Name(cluster=w282, "Clone"=w277) -> (w281:T8)
        n124 = case shown="False" w277 {
          tunnel: w280 -> [w285 w288]
          tunnel: [w284 w288] -> w279
          tunnel: w278 -> [w283 _]
          frame False {
            # "Initiate the VISA Resource selection window if this is not a"
            n125 = call "Enqueue Message (Single).vi"("error in (no error)"=w285, "Message Data"=refnum<visa-resource-name> refnum ("VISA resource out"), "Message"="Set VISA Resource", "Message Queue"=w283) -> ("error out"=w284:errorcluster)  [unwired: 6 in, 1 out]
          }
          frame True {
            # "Reentrant clone. It is the responsibility of the RCM to send the Set VISA Resource command."
          }
        }
      }
      frame "Error" {
        # "#CodeRecommended - If you ever change the name of this \"Error\" message, you'll need to update the name in the Check Loop Error.vi as well."
        # "#CodeRecommended - Consider creating a system for logging errors in some way. These errors are for notification purposes only. Handling of specific errors should be performed in the message frames that generated the error."
        # "Error - Display an error dialog. This message is sent by the \"Error Handler\" VIs at the end of other loops in this application."
        n126 = Variant To Data(error in=w295, type=errorcluster {"status"=FALSE, "code"=0, "source"=""} ("error constant"), Variant=w293) -> (data=w291:errorcluster, error out=w290:errorcluster)
        n127 = call <vilib>:"Simple Error Handler.vi"("error in (no error)"=w291) -> ()  [unwired: 4 in, 5 out]
        n128 = Merge Errors(w290) -> (w289:errorcluster)
      }
      frame "Confirm Quit" {
        # "#CodeNeeded - If you want to provide an \"Are you sure\" dialog (or some other notification) before the application exits, place that code here. This message is typically sent from a Panel Close? event."
        # "Confirm Quit - Message that can confirm whether or not the user wants to exit the application."
        n129 = call-poly "Enqueue Message.vi"("Priority Message? (F)"=TRUE, "error in (no error)"=w302, "Message"="Exit", "Message Queue"=w298) -> ("error out"=w299:errorcluster)  [unwired: 6 in, 1 out]
        n130 = Merge Errors(w299) -> (w300:errorcluster)
      }
      frame "Exit" {
        # "Order other processes to exit"
        # "Begin the application closing procedure by sending \"Exit\" commands to all running processes."
        n131 = Variant To Data(type=errorcluster {"status"=FALSE, "code"=0, "source"=""} ("error constant"), Variant=w322) -> (data=w323:errorcluster)  [unwired: 1 in, 1 out]
        n132 = Build Array(w312, w313, w316, w315, w314) -> (w311:refnum<queue>[])
        n133 = call <vilib>:"Clear Errors.vi"("error in (no error)"=w323, "specific error code to clear (0: all)"=5000) -> ("error out"=w304:errorcluster)  [unwired: 4 in, 1 out]
        n134 = call <vilib>:"Simple Error Handler.vi"("error in (no error)"=w304) -> ()  [unwired: 4 in, 5 out]
        n135 = for {
          tunnel: w318 -> [w329]
          tunnel: w311 -> [w328] mode=indexing
          shift-right: [w327] -> w320
          shift-left: _ -> [w326]
          n136 = call "Enqueue Message (Single).vi"("Priority Message? (F)"=TRUE, "Message"=w329, "Message Queue"=w328) -> ("error out"=w330:errorcluster)  [unwired: 7 in, 1 out]
          n137 = Merge Errors(w330, w326) -> (w327:errorcluster)
        }
        n138 = Release Notifier(notifier=w309) -> (error out=w308:errorcluster)  [unwired: 2 in, 2 out]
        n139 = Release Queue(queue=w307) -> (error out=w305:errorcluster)  [unwired: 2 in, 2 out]
        n140 = call "Fire User Event - Stop.vi"("User Event - Stop"=w319) -> ("error out"=w306:errorcluster)  [unwired: 10 in]
        n141 = Merge Errors(w306, w305, w308, w320) -> (w321:errorcluster)
      }
      frame Default {
        # "'Default' case only runs if there is a message that isn't defined in any of the other cases.  Output a programming error."
        n142 = xnode "Error Ring"("parameter 0"=w331) -> ("error out"=w332:errorcluster)
      }
      frame "---Copy This Frame---" {
        # "Sends the message to each process in the array."
        # "#CodeRecommended - Change connections to build an array of the processes that will receive this message"
        # "Duplicate this frame when creating new messages.  Change this comment in the duplicated frame to describe this message."
        n143 = Build Array(w348, w349, w350, w347, w346) -> (w343:refnum<queue>[])
        n144 = for {
          tunnel: w343 -> [w356] mode=indexing
          tunnel: w342 -> [w358]
          tunnel: w341 -> [w357]
          shift-right: [w355] -> w344
          shift-left: w345 -> [w353]
          n145 = call "Enqueue Message (Single).vi"("Message Data"=w357, "Message"=w358, "Message Queue"=w356) -> ("error out"=w354:errorcluster)  [unwired: 7 in, 1 out]
          n146 = Merge Errors(w354, w353) -> (w355:errorcluster)
        }
        n147 = Merge Errors(w344) -> (w351:errorcluster)
      }
      frame "Update Pressure Units" {
        # "Sends the message to each process in the array."
        # "Change the pressure units."
        n148 = Build Array(w359, w360) -> (w363:refnum<queue>[])
        n149 = for {
          tunnel: w363 -> [w371] mode=indexing
          tunnel: w362 -> [w373]
          tunnel: w361 -> [w372]
          shift-right: [w370] -> w364
          shift-left: w365 -> [w368]
          n150 = call "Enqueue Message (Single).vi"("Message Data"=w372, "Message"=w373, "Message Queue"=w371) -> ("error out"=w369:errorcluster)  [unwired: 7 in, 1 out]
          n151 = Merge Errors(w369, w368) -> (w370:errorcluster)
        }
        n152 = Merge Errors(w364) -> (w366:errorcluster)
      }
      frame "Update Flow Rate Units" {
        # "Sends the message to each process in the array."
        # "Change the flow rate units."
        n153 = Build Array(w374, w375) -> (w378:refnum<queue>[])
        n154 = for {
          tunnel: w378 -> [w386] mode=indexing
          tunnel: w377 -> [w388]
          tunnel: w376 -> [w387]
          shift-right: [w385] -> w379
          shift-left: w380 -> [w383]
          n155 = call "Enqueue Message (Single).vi"("Message Data"=w387, "Message"=w388, "Message Queue"=w386) -> ("error out"=w384:errorcluster)  [unwired: 7 in, 1 out]
          n156 = Merge Errors(w384, w383) -> (w385:errorcluster)
        }
        n157 = Merge Errors(w379) -> (w381:errorcluster)
      }
      frame "Set Remote Queue" {
        # "Sends the message to each process in the array."
        # "Bounce this message back to the Remote Control Manager to set the remote queue to publish messages to."
        n158 = Build Array(w394) -> (w391:refnum<queue>[])
        n159 = for {
          tunnel: w391 -> [w400] mode=indexing
          tunnel: w390 -> [w402]
          tunnel: w389 -> [w401]
          shift-right: [w399] -> w392
          shift-left: w393 -> [w397]
          n160 = call "Enqueue Message (Single).vi"("Message Data"=w401, "Message"=w402, "Message Queue"=w400) -> ("error out"=w398:errorcluster)  [unwired: 7 in, 1 out]
          n161 = Merge Errors(w398, w397) -> (w399:errorcluster)
        }
        n162 = Merge Errors(w392) -> (w395:errorcluster)
      }
      frame "Set VISA Resource" {
        # "Update the VISA Resource of the instrument."
        n163 = call "Enqueue Message (Single).vi"("error in (no error)"=w408, "Message Data"=w403, "Message"=w404, "Message Queue"=w405) -> ("error out"=w406:errorcluster)  [unwired: 6 in, 1 out]
        n164 = Merge Errors(w406) -> (w409:errorcluster)
      }
      frame "Valid VISA Resource" {
        # "When a Valid VISA Resource has been chosen, start the other processes."
        n165 = Unbundle By Name(w416) -> ("Log Runs"=w415:bool)
        n166 = call "Enqueue Message (Single).vi"("error in (no error)"=w426, "Message Data"=w411, "Message"=w410, "Message Queue"=w413) -> ("error out"=w414:errorcluster, "dup Message Queue"=w412:refnum<queue>)  [unwired: 6 in]
        n167 = case shown="True" w415 {
          tunnel: w414 -> [w427 w431]
          tunnel: w412 -> [_ w430]
          tunnel: [w427 w428] -> w424
          frame False {
          }
          frame True {
            n168 = call "Enqueue Message (Single).vi"("error in (no error)"=w431, "Message"="Start", "Message Queue"=w430) -> ("error out"=w428:errorcluster)  [unwired: 7 in, 1 out]
          }
        }
        n169 = call "Enqueue Message (Single).vi"("error in (no error)"=w424, "Message"="Start", "Message Queue"=w423) -> ("error out"=w422:errorcluster)  [unwired: 7 in, 1 out]
        n170 = Unbundle By Name(w416) -> ("Clone"=w418:bool)
        n171 = call "Enqueue Message (Single).vi"("error in (no error)"=w422, "Message Data"=w411, "Message"=w410, "Message Queue"=w421) -> ("error out"=w419:errorcluster)  [unwired: 6 in, 1 out]
        n172 = case shown="False" w418 {
          tunnel: w419 -> [w435 w436]
          tunnel: [w434 w436] -> w417
          tunnel: w420 -> [w433 _]
          frame False {
            # "Show the Front Panel automatically on startup"
            n173 = call "Enqueue Message (Single).vi"("error in (no error)"=w435, "Message"="Show", "Message Queue"=w433) -> ("error out"=w434:errorcluster)  [unwired: 7 in, 1 out]
          }
          frame True {
            # "Reentrant clone. It is the responsibility of the RCM to send \"Show\"."
          }
        }
      }
      frame "Logging" {
        # "Enable or disable logging in the System Data. Run logging is disabled by default."
        n174 = Variant To Data(type=TRUE, Variant=w441) -> (data=w440:bool)  [unwired: 1 in, 1 out]
        n175 = case shown="True" w440 {
          tunnel: w439 -> [w450 w455]
          tunnel: [w449 w454] -> w438
          tunnel: w437 -> [w448 w453]
          frame False {
            n176 = call "Enqueue Message (Single).vi"("Priority Message? (F)"=TRUE, "error in (no error)"=w450, "Message"="Stop", "Message Queue"=w448) -> ("error out"=w449:errorcluster)  [unwired: 6 in, 1 out]
          }
          frame True {
            n177 = call "Enqueue Message (Single).vi"("Priority Message? (F)"=TRUE, "error in (no error)"=w455, "Message"="Start", "Message Queue"=w453) -> ("error out"=w454:errorcluster)  [unwired: 6 in, 1 out]
          }
        }
        n178 = Bundle By Name(cluster=w445, "Log Runs"=w440) -> (w443:T8)
        n179 = Merge Errors(w438) -> (w444:errorcluster)
      }
      frame "Config Logging" {
        # "Pass on Config Logging message to Logging Loop."
        n180 = call "Enqueue Message (Single).vi"("error in (no error)"=w460, "Message Data"=w457, "Message"=w456, "Message Queue"=w458) -> ("error out"=w459:errorcluster)  [unwired: 6 in, 1 out]
        n181 = Merge Errors(w459) -> (w461:errorcluster)
      }
      frame "Set Log Directory" {
        # "Pass on log setting message to Logging Loop."
        n182 = call "Enqueue Message (Single).vi"("error in (no error)"=w467, "Message Data"=w464, "Message"=w463, "Message Queue"=w465) -> ("error out"=w466:errorcluster)  [unwired: 6 in, 1 out]
        n183 = Merge Errors(w466) -> (w468:errorcluster)
      }
      frame "Set Log File Prefix" {
        # "Pass on log setting message to Logging Loop."
        n184 = call "Enqueue Message (Single).vi"("error in (no error)"=w474, "Message Data"=w471, "Message"=w470, "Message Queue"=w472) -> ("error out"=w473:errorcluster)  [unwired: 6 in, 1 out]
        n185 = Merge Errors(w473) -> (w475:errorcluster)
      }
      frame "Set Log File Delimiter" {
        # "Pass on log setting message to Logging Loop."
        n186 = call "Enqueue Message (Single).vi"("error in (no error)"=w481, "Message Data"=w478, "Message"=w477, "Message Queue"=w479) -> ("error out"=w480:errorcluster)  [unwired: 6 in, 1 out]
        n187 = Merge Errors(w480) -> (w482:errorcluster)
      }
      frame "Set Log on Run" {
        # "Pass on log setting message to Logging Loop."
        n188 = call "Enqueue Message (Single).vi"("error in (no error)"=w488, "Message Data"=w485, "Message"=w484, "Message Queue"=w486) -> ("error out"=w487:errorcluster)  [unwired: 6 in, 1 out]
        n189 = Merge Errors(w487) -> (w489:errorcluster)
      }
      frame "Logging Started" {
        # "Pass on Logging Started message to RCM and UI."
        n190 = Build Array(w492, w493) -> (w491:refnum<queue>[])
        n191 = for {
          tunnel: w495 -> [w502]
          tunnel: w494 -> [w501]
          shift-right: [w503] -> w496
          shift-left: w497 -> [w504]
          tunnel: w491 -> [w500] mode=indexing
          n192 = call "Enqueue Message (Single).vi"("error in (no error)"=w504, "Message Data"=w502, "Message"=w501, "Message Queue"=w500) -> ("error out"=w503:errorcluster)  [unwired: 6 in, 1 out]
        }
        n193 = Merge Errors(w496) -> (w498:errorcluster)
      }
      frame "Logging Stopped" {
        # "Pass on Logging Stopped message to RCM and UI."
        n194 = Build Array(w506, w507) -> (w505:refnum<queue>[])
        n195 = for {
          tunnel: w509 -> [w516]
          tunnel: w508 -> [w515]
          shift-right: [w517] -> w510
          shift-left: w511 -> [w518]
          tunnel: w505 -> [w514] mode=indexing
          n196 = call "Enqueue Message (Single).vi"("error in (no error)"=w518, "Message Data"=w516, "Message"=w515, "Message Queue"=w514) -> ("error out"=w517:errorcluster)  [unwired: 6 in, 1 out]
        }
        n197 = Merge Errors(w510) -> (w512:errorcluster)
      }
      frame "Change Refresh" {
        # "#CodeRecommended - If the default refresh time is changed, it must be updated in the UI and Data Acquisition Loop Data typedef."
        # "Change the sampling rate of the instrument. Default is 1 second/sample."
        n198 = Build Array(w520, w521) -> (w519:refnum<queue>[])
        n199 = for {
          tunnel: w523 -> [w530]
          tunnel: w522 -> [w529]
          tunnel: w519 -> [w528] mode=indexing
          shift-right: [w531] -> w524
          shift-left: w527 -> [w532]
          n200 = call "Enqueue Message (Single).vi"("error in (no error)"=w532, "Message Data"=w529, "Message"=w530, "Message Queue"=w528) -> ("error out"=w531:errorcluster)  [unwired: 6 in, 1 out]
        }
        n201 = Merge Errors(w524) -> (w525:errorcluster)
      }
      frame "Change Flow Rate" {
        # "Forward the Change Setpoint command to the IML and acquisition."
        n202 = Build Array(w534, w535) -> (w533:refnum<queue>[])
        n203 = for {
          tunnel: w537 -> [w544]
          tunnel: w536 -> [w543]
          shift-right: [w545] -> w538
          shift-left: w541 -> [w546]
          tunnel: w533 -> [w542] mode=indexing
          n204 = call "Enqueue Message (Single).vi"("error in (no error)"=w546, "Message Data"=w543, "Message"=w544, "Message Queue"=w542) -> ("error out"=w545:errorcluster)  [unwired: 6 in, 1 out]
        }
        n205 = Merge Errors(w538) -> (w539:errorcluster)
      }
      frame "Update Total Flow Rate" {
        # "Forward the new total flow rate command to the IML and acquisition."
        n206 = Build Array(w548) -> (w547:refnum<queue>[])
        n207 = for {
          tunnel: w550 -> [w557]
          tunnel: w549 -> [w556]
          shift-right: [w558] -> w551
          shift-left: w554 -> [w559]
          tunnel: w547 -> [w555] mode=indexing
          n208 = call "Enqueue Message (Single).vi"("error in (no error)"=w559, "Message Data"=w556, "Message"=w557, "Message Queue"=w555) -> ("error out"=w558:errorcluster)  [unwired: 6 in, 1 out]
        }
        n209 = Merge Errors(w551) -> (w552:errorcluster)
      }
      frame "Start Instrument" {
        # "Pass message to Instrument Manager Loop."
        n210 = call "Enqueue Message (Single).vi"("error in (no error)"=w564, "Message Data"=w562, "Message"=w561, "Message Queue"=w560) -> ("error out"=w563:errorcluster)  [unwired: 6 in, 1 out]
        n211 = Merge Errors(w563) -> (w565:errorcluster)
      }
      frame "Stop Instrument" {
        # "Pass message to Instrument Manager Loop."
        n212 = call "Enqueue Message (Single).vi"("error in (no error)"=w571, "Message Data"=w569, "Message"=w568, "Message Queue"=w567) -> ("error out"=w570:errorcluster)  [unwired: 6 in, 1 out]
        n213 = Merge Errors(w570) -> (w572:errorcluster)
      }
      frame "Instrument Started" {
        # "Build an array of all processes that will receive this message"
        # "Notify processes of update"
        # "Notify processes that the instrument is running."
        n214 = Build Array(w580, w575, w574) -> (w581:refnum<queue>[])
        n215 = for {
          tunnel: w581 -> [w585] mode=indexing
          tunnel: w578 -> [w587]
          tunnel: w579 -> [w586]
          shift-right: [w584] -> w577
          shift-left: _ -> [w582]
          n216 = call "Enqueue Message (Single).vi"("Message Data"=w586, "Message"=w587, "Message Queue"=w585) -> ("error out"=w583:errorcluster)  [unwired: 7 in, 1 out]
          n217 = Merge Errors(w583, w582) -> (w584:errorcluster)
        }
      }
      frame "Instrument Stopped" {
        # "Build an array of all processes that will receive this message"
        # "Notify processes of update"
        # "Notify processes that the instrument stopped running."
        n218 = Build Array(w588, w590) -> (w591:refnum<queue>[])
        n219 = for {
          tunnel: w591 -> [w598] mode=indexing
          tunnel: w593 -> [w600]
          tunnel: w594 -> [w599]
          shift-right: [w597] -> w592
          shift-left: _ -> [w595]
          n220 = call "Enqueue Message (Single).vi"("Message Data"=w599, "Message"=w600, "Message Queue"=w598) -> ("error out"=w596:errorcluster)  [unwired: 7 in, 1 out]
          n221 = Merge Errors(w596, w595) -> (w597:errorcluster)
        }
      }
      frame "Report" {
        # "Send instrument state notification"
        # "Notify processes that the instrument stopped running."
        n222 = Variant To Data(type=T2 {"VISA Resource"="", "Flow Rate"=0.0, "Running"=FALSE, "Running Since"=timestamp(0 s since 1904-01-01), "Pressure Data Point"={"Time Stamp"=timestamp(0 s since 1904-01-01), "Value"=0.0}, "Upper Pressure Fault"=FALSE, "Lower Pressure Fault"=FALSE, "Motor Stall Fault"=FALSE, "Sampling Rate (sec/sample)"=0.0, "Retry Attempts"=0, "Fast Comms"=FALSE, "Total Flow Rate"=0.0, "Other Flow Rate"=0.0} ("Instrument State"), Variant=w610) -> (data=w606:T2)  [unwired: 1 in, 1 out]
        n223 = local read "Sampling rate\n(sec/sample)"() -> (w602:dbl)
        n224 = Bundle By Name(cluster=w606, "Sampling Rate (sec/sample)"=w602) -> (w601:T2)
        n225 = Enqueue Element(queue=w607, element=w601) -> (error out=w604:errorcluster)  [unwired: 2 in, 2 out]
        n226 = Send Notification(notification=w601, notifier=w611) -> (error out=w608:errorcluster)  [unwired: 1 in, 1 out]
        n227 = Merge Errors(w604, w608) -> (w605:errorcluster)
        n228 = call "Enqueue Message (Single).vi"("Message Data"=w601, "Message"=w615, "Message Queue"=w613) -> ("error out"=w603:errorcluster)  [unwired: 7 in, 1 out]
        n229 = Merge Errors(w603, w605) -> (w614:errorcluster)
      }
    }
    n230 = call "Error Handler - System Control Loop.vi"("error in (no error)"=w265, "Message Queue"=w267) -> ("dup error in"=w266:errorcluster)  [unwired: 8 in, 1 out]
  }
  n231 = call "Logging Message Loop.vi"("System Control"=w4, "Data Queue"=w6, "Logging"=w31) -> ("error out"=w16:errorcluster)  [unwired: 8 in]
  n232 = Unregister For Events(event registration refnum=w23) -> (error out=w18:errorcluster)  [unwired: 1 in]
  n233 = Merge Errors(w27, w19, w18, w17, w16, w15, w14) -> (w12:errorcluster)
  n234 = call <vilib>:"Simple Error Handler.vi"("error in (no error)"=w12) -> ()  [unwired: 4 in, 5 out]
  n235 = Cluster To Array(cluster=w11) -> (array=w10:refnum<queue>[])
  n236 = for {
    shift-right: [w617] -> w9
    shift-left: w12 -> [w618]
    tunnel: w10 -> [w619] mode=indexing
    n237 = Release Queue(queue=w619, force destroy? (F)=TRUE, error in (no error)=w618) -> (error out=w617:errorcluster)  [unwired: 2 out]
  }
  n238 = call "Destroy User Event - Stop.vi"("error in (no error)"=w9, "User Event - Stop"=w22) -> ("error out"=w24:errorcluster)  [unwired: 9 in]
  n239 = disable-structure shown="RUN_TIME_ENGINE==True" {
    disable-tunnel: w24 -> [_ _]
    frame condition #0 (active) {
    }
    frame condition #1 {
      # "Call Quit LabVIEW if running as a built application."
      n240 = Quit LabVIEW() -> ()  [unwired: 1 in]
    }
  }
